vi "QL355P_voltage_source.vi"() -> ()   [LabVIEW 2012]
panel:
  in  "Boolean":bool
  out "set V [V]":string
  in  "V [V]":string
  in  "Keithley":refnum<visa-resource-name>="GPIB1::20::INSTR"
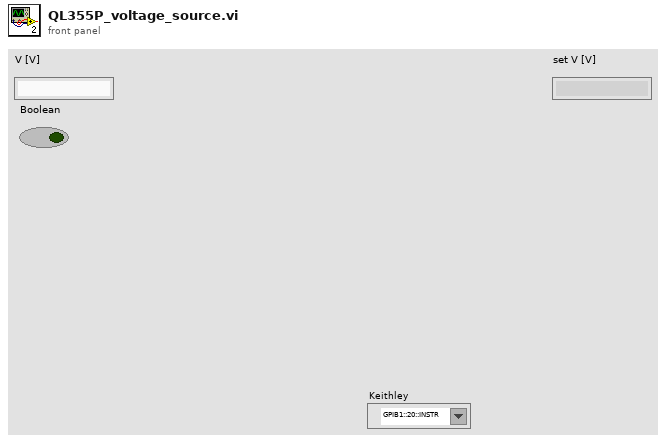
[diagram p1: front panel]
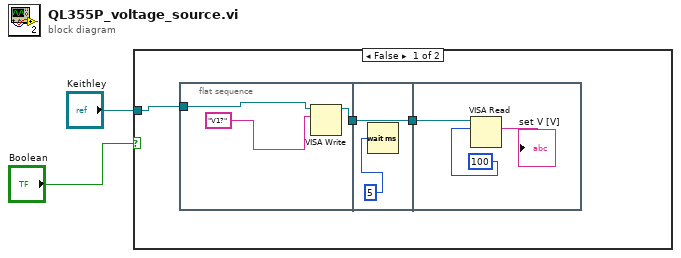
[diagram p0: block diagram]
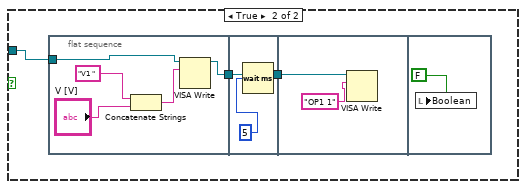
[diagram p2: hidden frame]
diagram:
  n1 = case shown="False" "Boolean" {
    tunnel: "Keithley" -> [w5 w16]
    frame False {
      n2 = flat-sequence {
        tunnel: w5 -> [w8]
        tunnel: [w6] -> w3
        tunnel: [w10] -> w4
        tunnel: w3 -> [w10]
        tunnel: w4 -> [w13]
        frame #0 {
          n3 = VISA Write(VISA resource name=w8, write buffer="V1?" ("write buffer 2")) -> (VISA resource name out=w6:refnum<visa-resource-name>)  [unwired: 1 in, 2 out]
        }
        frame #1 {
          n4 = Wait (ms)(milliseconds to wait=u32 5) -> ()  [unwired: 1 out]
        }
        frame #2 {
          n5 = VISA Read(VISA resource name=w13, byte count=u32 100) -> (read buffer=→"set V [V]":string)  [unwired: 1 in, 3 out]
        }
      }
    }
    frame True {
      n6 = flat-sequence {
        tunnel: w16 -> [w21]
        tunnel: [w17] -> w15
        tunnel: w15 -> [w23]
        tunnel: [w23] -> w14
        tunnel: w14 -> [w25]
        frame #0 {
          n7 = Concatenate Strings("V1 " ("write buffer 2"), "V [V]") -> (w18:string)
          n8 = VISA Write(VISA resource name=w21, write buffer=w18) -> (VISA resource name out=w17:refnum<visa-resource-name>)  [unwired: 1 in, 2 out]
        }
        frame #1 {
          n9 = Wait (ms)(milliseconds to wait=u32 5) -> ()  [unwired: 1 out]
        }
        frame #2 {
          n10 = VISA Write(VISA resource name=w25, write buffer="OP1 1" ("write buffer 2")) -> ()  [unwired: 1 in, 3 out]
        }
        frame #3 {
          n11 = local write "Boolean"(FALSE) -> ()
        }
      }
    }
  }
